vi "Configure Voltage Level.vi"(8 "error in (no error)":errorcluster, 9 "level (0.0 Volts)":dbl[unit] format="%^.2e", 10 "channel name (\"CHANNEL1\")":string="CHANNEL1", 11 "CS++DCPwr in":refnum<class "CS++DCPwr.lvclass">) -> (0 "error out":errorcluster, 3 "CS++DCPwr out":refnum<class "CS++DCPwr.lvclass">)   [LabVIEW 2013, in "CS++DCPwr.lvlib" / "CS++DCPwr.lvclass"]
doc: "This VI configures the DC voltage level that the power supply attempts to generate."
uses:
  CS++DCPwr.lvclass
  CSPP_Core/Classes/CS++ProcessVariables/ProcessVariable/PV.lvclass
  CSPP_Core/Classes/CS++ProcessVariables/ProcessVariable/PV.lvclass/PV.ctl
  CS++DCPwr.lvclass/CS++DCPwr.ctl
  CSPP_Core/Classes/CS++ProcessVariables/PVConnection/PVConnection.lvclass
  CSPP_Core/Classes/CS++ProcessVariables/ProcessVariable/Write Data.vi
  CSPP_Core/Classes/CS++ProcessVariables/ProcessVariable/Write Timestamp.vi
  CSPP_Core/Classes/CS++ProcessVariables/ProcessVariable/Write Quality.vi
  CSPP_Core/Classes/CS++ProcessVariables/ProcessVariable/Write status.vi
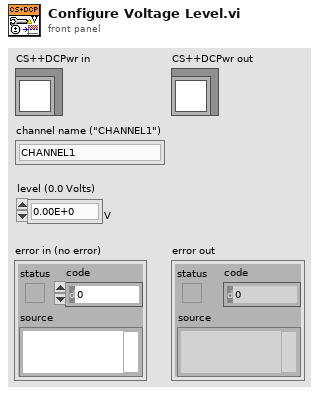
[diagram p1: front panel]
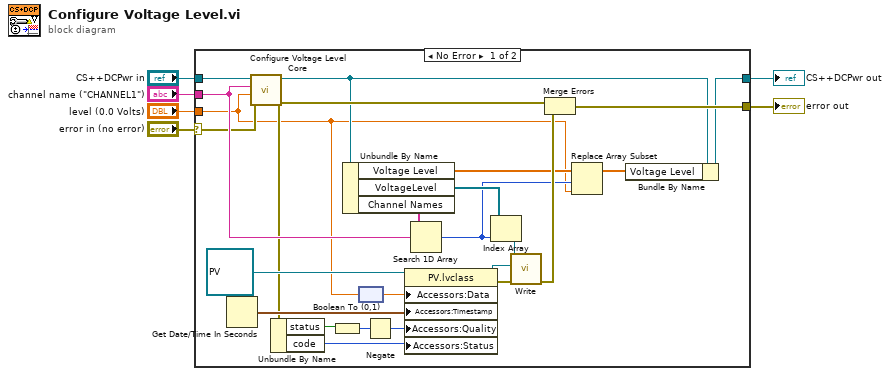
[diagram p0: block diagram]
diagram:
  n1 = case shown="No Error" "error in (no error)" {
    selector: "error in (no error)" -> [w9 w31]
    tunnel: "CS++DCPwr in" -> [w30 w32]
    tunnel: "level (0.0 Volts)" -> [w8 _]
    tunnel: "channel name (\"CHANNEL1\")" -> [w17 _]
    tunnel: [w15 w31] -> w4
    tunnel: [w13 w32] -> w5
    frame No Error {
      n2 = Get Date/Time In Seconds() -> (seconds since 1Jan1904=w29:timestamp)
      n3 = call-dynamic "Configure Voltage Level Core.vi"("error in (no error)"=w9, "level (0.0 Volts)"=w8, "channel name (\"CHANNEL1\")"=w17, "CS++DCPwr in"=w30) -> ("error out"=w16:errorcluster, "CS++DCPwr out"=w14:refnum<class "CS++DCPwr.lvclass">)  [unwired: 6 in]
      n4 = Unbundle By Name(w16) -> ("status"=w21:bool, "code"=w19:i32)
      n5 = Boolean To (0,1)(Boolean=w21) -> (0, 1=w20:i16)
      n6 = Unbundle By Name(w14) -> ("Voltage Level"=w12:dbl[unit][], "VoltageLevel"=w24:refnum<class "PVConnection.lvclass">[], "Channel Names"=w25:string[])
      n7 = node(w8) -> (w7:dbl)
      n8 = Negate(x=w20) -> (-x=w18:i16)
      n9 = property class="PV.lvclass"(reference=refnum<class "PV.lvclass"> refnum ("PV"), "Accessors:Data"=w7, "Accessors:Timestamp"=w29, "Accessors:Quality"=w18, "Accessors:Status"=w19) -> (reference out=w26:refnum<class "PV.lvclass">, error out=w27:errorcluster)  [unwired: 1 in]
      n10 = Search 1D Array(1D array=w25, element=w17) -> (index of element=w10:i32)  [unwired: 1 in]
      n11 = Index Array(array=w24, index=w10) -> (element=w23:refnum<class "PVConnection.lvclass">)
      n12 = call-dynamic "Write.vi"("error in (no error)"=w27, "PV"=w26, "PVConnection in"=w23) -> ("error out"=w22:errorcluster)  [unwired: 7 in, 1 out]
      n13 = Merge Errors(w16, w22) -> (w15:errorcluster)
      n14 = Replace Array Subset(array=w12, new element=w8, index=w10) -> (w11:dbl[unit][])
      n15 = Bundle By Name(cluster=w14, "Voltage Level"=w11) -> (w13:refnum<class "CS++DCPwr.lvclass">)
    }
    frame Error {
    }
  }
  "error out" <- w4
  "CS++DCPwr out" <- w5
